vi "报文数据拆分.vi"(0 "字符串":string="##QN=1;GO=1;CP=&&address=192.168.16.237,username=cc,password=std23506,filename=一体化微型水质监测站.exe,localpath=C:\\Users\\Administrator\\Desktop\\ftp接收文件\\一体化微型水质监测站.exe&&\r\n") -> (3 "filename":string, 4 "QN":string, 6 "GO":string, 8 "address":string, 10 "username":string, 14 "localpath":string, 15 "password":string)   [LabVIEW 2016]
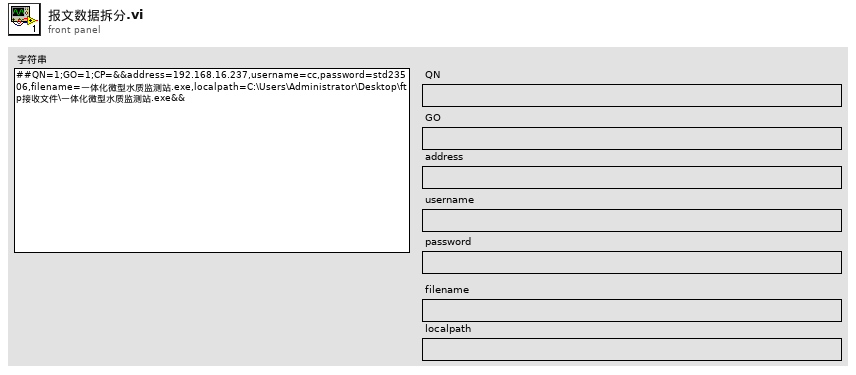
[diagram p1: front panel]
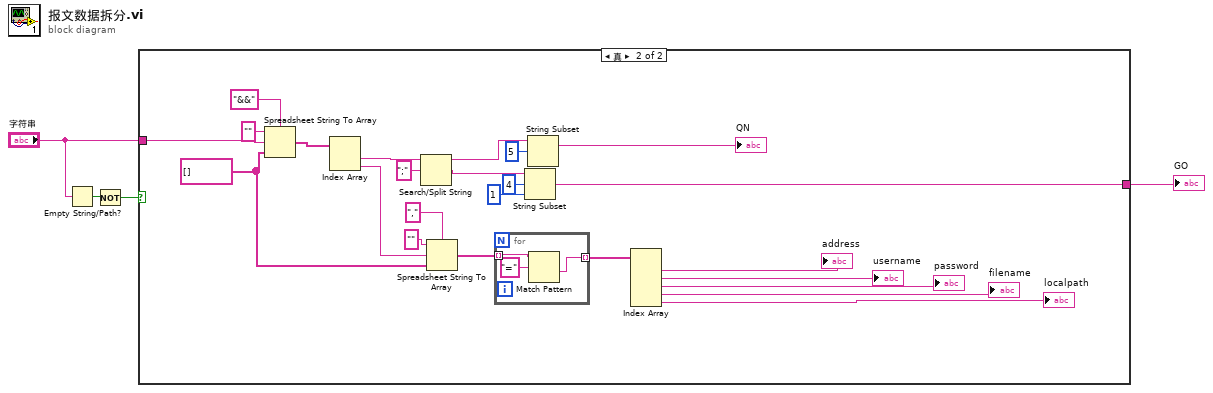
[diagram p0: block diagram]
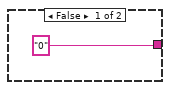
[diagram p2: hidden frame]
diagram:
  n1 = Empty String/Path?(string/path="字符串") -> (empty?=w4:bool)
  n2 = Not(x=w4) -> (.not. x?=w3:bool)
  n3 = case shown="真" w3 {
    tunnel: "字符串" -> [_ w29]
    tunnel: ["0" ("GO") w6] -> w1
    frame False {
    }
    frame True {
      w14 = string[] [] ("数组 2")
      n4 = Spreadsheet String To Array(delimiter (Tab)="&&" ("分隔符(Tab)"), format string="" ("格式字符串"), spreadsheet string=w29, array type (2D Dbl)=w14) -> (array=w26:string[])
      n5 = Index Array(array=w26) -> (element #1=w25:string, element #2=w16:string)  [unwired: 2 in]
      n6 = Search/Split String(string=w25, search string/char (-)=";" ("搜索字符串/字符(-)")) -> (substring before match=w24:string, match + rest of string=w21:string)  [unwired: 1 in, 1 out]
      n7 = Spreadsheet String To Array(delimiter (Tab)="," ("分隔符(Tab)"), format string="" ("格式字符串"), spreadsheet string=w16, array type (2D Dbl)=w14) -> (array=w8:string[])
      n8 = for {
        tunnel: w8 -> [w32] mode=indexing
        tunnel: [w30] -> w7 mode=indexing
        n9 = Match Pattern(string=w32, regular expression="=" ("正则表达式")) -> (after substring=w30:string)  [unwired: 1 in, 3 out]
      }
      n10 = String Subset(string=w21, offset (0)=4 ("偏移量(0)"), length (rest)=1 ("长度（剩余）")) -> (substring=w6:string)
      n11 = String Subset(string=w24, offset (0)=5 ("偏移量(0)")) -> (substring=→"QN":string)  [unwired: 1 in]
      n12 = Index Array(array=w7) -> (element #1=→"address":string, element #2=→"username":string, element #3=→"password":string, element #4=→"filename":string, element #5=→"localpath":string)  [unwired: 5 in]
    }
  }
  "GO" <- w1
